vi "Echo_Register.vi"(7 "I2C Channel":u8, 8 "error in (no error)":errorcluster, 10 "Register to Echo":u8(ring) items=["CTRL_REG1"=32, "CTRL_REG2"=33, "CTRL_REG3"=34, "CTRL_REG4"=35, "CTRL_REG5"=36, "HP_FILTER_RESET"=37, "REFERENCE"=38, "STATUS_REG"=39, "OUT_X_L"=40, "OUT_X_H"=41, "OUT_Y_L"=42, "OUT_Y_H"=43, "OUT_Z_L"=44, "OUT_Z_H"=45, "INT1_CFG"=48, "INT1_SOURCE"=49, "INT1_THS"=50, "INT1_DURATION"=51, "INT2_CFG"=52, "INT2_SOURCE"=53, "INT2_THS"=54, "INT2_DURATION"=55], 11 "LINX Resource In":T1) -> (0 "error out":errorcluster, 2 "Register Word":u8 format="%x", 3 "LINX Resource Out":T1)   [LabVIEW 2014, in "LMH-LINX.lvlib" / "LIS331HH.lvlib"]
doc: "This VI isused to echo the contents of the specified register. \n\n**Author: Stas Legedza"
uses:
  <vilib>/MakerHub/LINX/Public/Sensors/Accelerometer/LIS331HH/LIS331HH.lvlib
  <vilib>/MakerHub/LINX/Private/Type Defs/LINX Ref.ctl
  <vilib>/MakerHub/LINX/Private/Type Defs/Platform.ctl
  <vilib>/MakerHub/LINX/Private/Type Defs/Interface.ctl
  <vilib>/MakerHub/LINX/Private/Device/Type Defs/LINX Device Config.ctl
  <vilib>/MakerHub/LINX/Private/Device/Type Defs/TCP Config.ctl
  <vilib>/MakerHub/LINX/Private/Device/Type Defs/Channels.ctl
  <vilib>/MakerHub/LINX/Private/Local IO/LinxI2cWrite.vi
  <vilib>/MakerHub/LINX/Public/Utilities/Check Channel.vi
  <vilib>/MakerHub/LINX/Private/Utilties/Generate Error.vi
  <vilib>/MakerHub/LINX/LMH-LINX.lvlib
  <vilib>/MakerHub/LINX/Private/Device/Device.lvlib
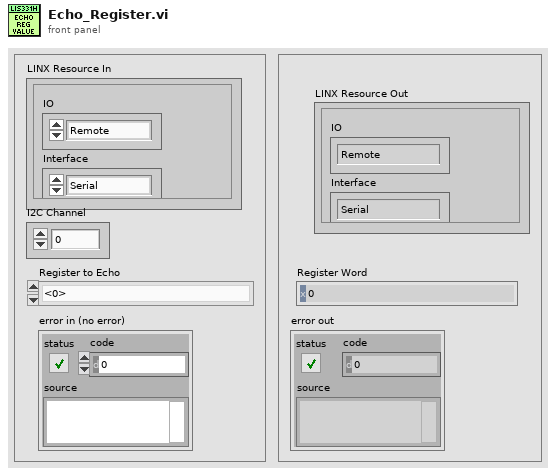
[diagram p1: front panel]
types:
  T1 = typedef "LMH-LINX.lvlib/LINX Ref.ctl" = cluster{"IO":T2, "Interface":T3, "LINX Device Config":T4}
  T2 = typedef "LMH-LINX.lvlib/Platform.ctl" = enum16{"Remote", "Local"}
  T3 = typedef "LMH-LINX.lvlib/Interface.ctl" = enum16{"Serial", "TCP"}
  T4 = typedef "LMH-LINX.lvlib/Device.lvlib/LINX Device Config.ctl" = cluster{"Interface":T3, "COM Port":refnum<visa-resource-name>, "TCP Configuration":T5, "Device Family":u8, "Device ID":u8, "Device Name":string, "TCP Ref":refnum<k5>, "Channels":T6}
  T5 = typedef "LMH-LINX.lvlib/Device.lvlib/TCP Config.ctl" = cluster{"IP Address":string, "Port":u16}
  T6 = typedef "LMH-LINX.lvlib/Channels.ctl" = cluster{"DI":u8[], "DO":u8[], "AI":u8[], "AO":u8[], "PWM":u8[], "QE":u8[], "UART":u8[], "I2C 2":u8[], "SPI":u8[], "CAN":u8[], "Servo":u8[], "AI Ref (V)":dbl, "AI Resolution (Bits)":u8, "AO Ref (V)":dbl, "AO Resolution (Bits)":u8}
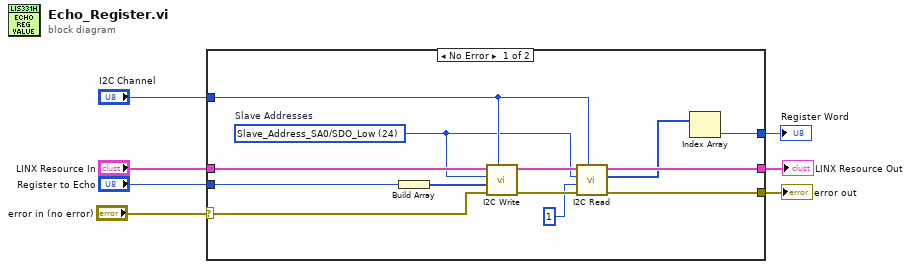
[diagram p0: block diagram]
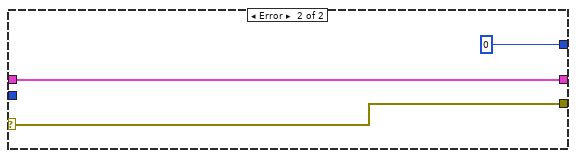
[diagram p2: hidden frame]
diagram:
  n1 = case shown="No Error" "error in (no error)" {
    selector: "error in (no error)" -> [w19 w23]
    tunnel: [w18 w23] -> w6
    tunnel: "LINX Resource In" -> [w20 w22]
    tunnel: "I2C Channel" -> [w16 _]
    tunnel: [w17 w22] -> w3
    tunnel: "Register to Echo" -> [w10 _]
    tunnel: [w8 u8 0 ("element")] -> w1
    frame No Error {
      w9 = u8 24 items=["Slave_Address_SA0/SDO_Low"=24, "Slave_Address_SA0/SDO_High"=25]  # Slave Addresses
      n2 = Build Array(w10) -> (w15:u8[])
      n3 = call <vilib>:"I2C Write.vi"("I2C Channel"=w16, "Error In"=w19, "Data"=w15, "I2C Slave Address (0)"=w9, "LINX Resource"=w20) -> ("Error Out"=w13:errorcluster, "LINX Resource"=w14:T1)  [unwired: 5 in]
      n4 = call <vilib>:"I2C Read.vi"("I2C Channel"=w16, "Error In"=w13, "Bytes To Read"=u8 1, "I2C Slave Address (0)"=w9, "LINX Resource"=w14) -> ("Error Out"=w18:errorcluster, "Data"=w11:u8[], "LINX Resource"=w17:T1)  [unwired: 4 in]
      n5 = Index Array(array=w11) -> (element=w8:u8)  [unwired: 1 in]
    }
    frame Error {
    }
  }
  "error out" <- w6
  "LINX Resource Out" <- w3
  "Register Word" <- w1
